vi "2019-05-07_3.vi"() -> ()   [LabVIEW 2018]
panel:
  in  "배열":dbl[](array[numeric])
  out "Result String":string
  out "Length":dbl
  in  "Unit":string
  in  "C":string
  out "Voltage meter":dbl(knob) scale=0.0..10.0
  out "Current meter":dbl(knob) scale=0.0..10.0
  in  "B":string
  in  "A":string
  out "Date / Time":string
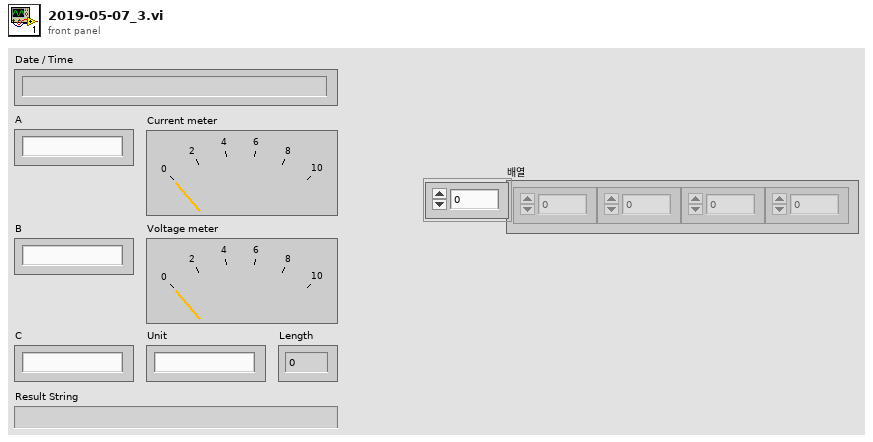
[diagram p1: front panel]
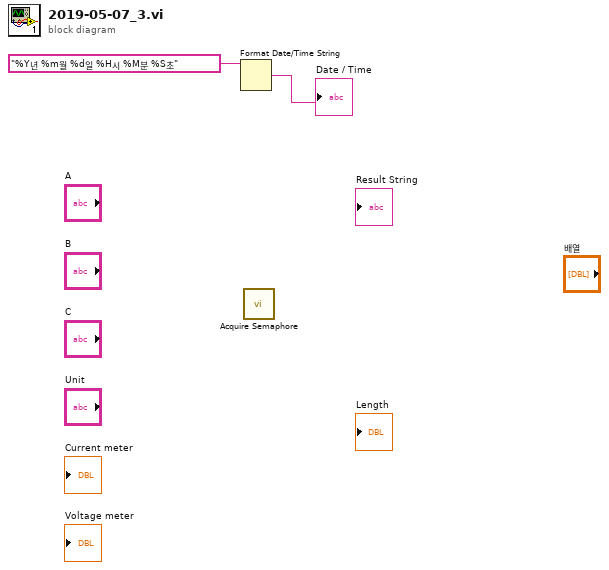
[diagram p0: block diagram]
diagram:
  n1 = Format Date/Time String(time format string (%c)="%Y년 %m월 %d일 %H시 %M분 %S초") -> (date/time string=→"Date / Time":string)  [unwired: 2 in]
  n2 = call <vilib>:"Acquire Semaphore.vi"() -> ()  [unwired: 5 in, 3 out]
